vi "Next.vi"(0 "object in":refnum<class "DFSTreeIterator.lvclass">, 5 "Error In":errorcluster) -> (14 "object out":refnum<class "DFSTreeIterator.lvclass">, 16 "Next":refnum<class "Element.lvclass">, 19 "Error Out":errorcluster)   [LabVIEW 2024, in "DFSTreeIterator.lvclass"]
uses:
  DFSTreeIterator.lvclass
  Element_interface/Element.lvclass
  Node_class/Node.lvclass
  C:/Users/burakkorkmaz/Desktop/Leveling/labview-desing-patterns/Iterator Pattern/Element_interface/Element.lvclass
  DFSTreeIterator.lvclass/DFSTreeIterator.ctl
  Support/Stack_class/Stack.lvclass
panel:
  # "Connector Pane"
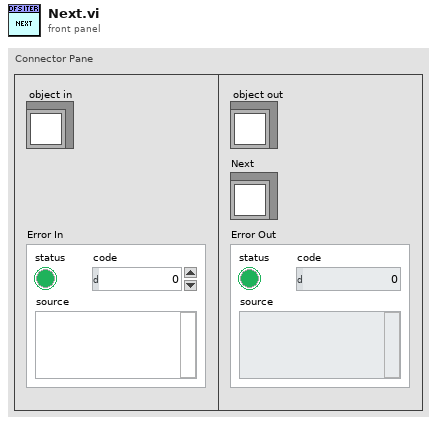
[diagram p1: front panel]
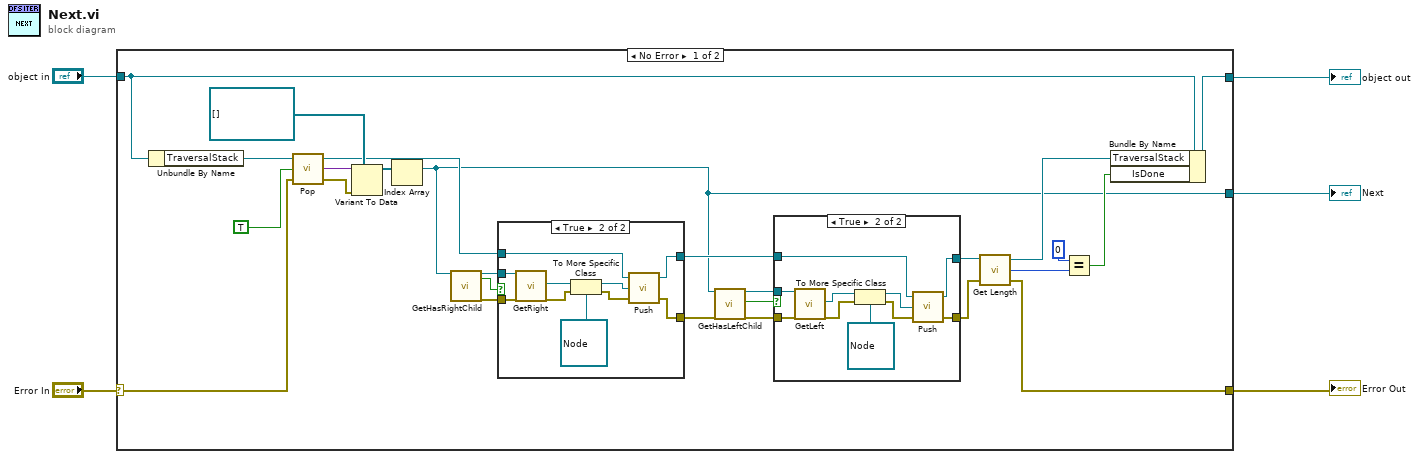
[diagram p0: block diagram]
diagram:
  n1 = case shown="No Error" "Error In" {
    selector: "Error In" -> [w14 w57]
    tunnel: [w13 w57] -> w2
    tunnel: [w23 w56] -> w3
    tunnel: "object in" -> [w31 w56]
    tunnel: [w7 _] -> w1
    frame No Error {
      n2 = Unbundle By Name(w31) -> ("TraversalStack"=w30:refnum<class "Stack.lvclass">)
      n3 = call-dynamic "Pop.vi"("Error In"=w14, "Delete?"=TRUE, "object in"=w30) -> ("Error Out"=w27:errorcluster, "Data"=w29:variant, "object out"=w22:refnum<class "Stack.lvclass">)
      n4 = Variant To Data(error in=w27, type=refnum<class "Node.lvclass">[] [] ("Array"), Variant=w29) -> (data=w20:refnum<class "Node.lvclass">[])  [unwired: 1 out]
      n5 = Index Array(array=w20) -> (element=w7:refnum<class "Node.lvclass">)  [unwired: 1 in]
      n6 = call-dynamic "GetHasRightChild.vi"("object in"=w7) -> ("object out"=w24:refnum<class "Node.lvclass">, "HasRightChild"=w26:bool, "Error Out"=w25:errorcluster)  [unwired: 16 in]
      n7 = case shown="True" w26 {
        tunnel: w22 -> [w45 w46]
        tunnel: w25 -> [w44 w55]
        tunnel: [w44 w54] -> w21
        tunnel: [w45 w53] -> w17
        tunnel: w24 -> [_ w48]
        frame False {
        }
        frame True {
          n8 = call-dynamic "GetRight.vi"("object in"=w48, "Error In"=w55) -> ("Right"=w49:refnum<class "Element.lvclass">, "Error Out"=w50:errorcluster)  [unwired: 15 in, 1 out]
          n9 = To More Specific Class(target class=refnum<class "Node.lvclass"> refnum ("Node"), reference=w49, error in=w50) -> (specific class reference=w47:refnum<class "Node.lvclass">, error out=w52:errorcluster)
          n10 = call-dynamic "Push.vi"("Error In"=w52, "Data"=w47, "object in"=w46) -> ("Error Out"=w54:errorcluster, "object out"=w53:refnum<class "Stack.lvclass">)  [unwired: 1 in]
        }
      }
      n11 = call-dynamic "GetHasLeftChild.vi"("object in"=w7, "Error In"=w21) -> ("object out"=w18:refnum<class "Node.lvclass">, "HasLeftChild"=w6:bool, "Error Out"=w19:errorcluster)  [unwired: 15 in]
      n12 = case shown="True" w6 {
        tunnel: w17 -> [w33 w43]
        tunnel: w19 -> [w32 w42]
        tunnel: [w32 w41] -> w15
        tunnel: [w33 w40] -> w16
        tunnel: w18 -> [_ w34]
        frame False {
        }
        frame True {
          n13 = call-dynamic "GetLeft.vi"("object in"=w34, "Error In"=w42) -> ("Left"=w35:refnum<class "Element.lvclass">, "Error Out"=w36:errorcluster)  [unwired: 15 in, 1 out]
          n14 = To More Specific Class(target class=refnum<class "Node.lvclass"> refnum ("Node"), reference=w35, error in=w36) -> (specific class reference=w38:refnum<class "Node.lvclass">, error out=w39:errorcluster)
          n15 = call-dynamic "Push.vi"("Error In"=w39, "Data"=w38, "object in"=w43) -> ("Error Out"=w41:errorcluster, "object out"=w40:refnum<class "Stack.lvclass">)  [unwired: 1 in]
        }
      }
      n16 = call-dynamic "Get Length.vi"("Error In"=w15, "object in"=w16) -> ("Error Out"=w13:errorcluster, "Length"=w12:i32, "object out"=w9:refnum<class "Stack.lvclass">)  [unwired: 1 in]
      n17 = Equal?(x=0, y=w12) -> (x = y?=w10:bool)
      n18 = Bundle By Name(cluster=w31, "TraversalStack"=w9, "IsDone"=w10) -> (w23:refnum<class "DFSTreeIterator.lvclass">)
    }
    frame Error {
    }
  }
  "Error Out" <- w2
  "object out" <- w3
  "Next" <- w1
